vi "Angle Vector to Rotation Matrix.vi"(1 "vector":dbl[](array[numeric]), 2 "angle":dbl) -> (0 "rotation matrix":dbl[][](array[numeric]))   [LabVIEW 2021]
doc: "This VI transforms angle vector to rotation matrix."
uses:
  <vilib>/Analysis/_algsub.llb/Real Vector Norm.vi
  <vilib>/Analysis/baseanly.llb/Real Outer Product.vi
  <vilib>/Analysis/7linalg.llb/Create Special Real Matrix.vi
  <vilib>/Analysis/Matrix/Numeric/Multiply/Multiply - RM,R.vi
  <vilib>/Analysis/Matrix/Numeric/Multiply/Multiply - R,RM.vi
  <vilib>/Analysis/Matrix/Numeric/Add/Add - RM,RM.vi
  <vilib>/Analysis/NI_AALPro.lvlib
  <vilib>/Analysis/NI_AALBase.lvlib
  <vilib>/Analysis/Matrix/NI_Matrix.lvlib
panel:
  # "This VI transforms angle vector to rotation matrix."
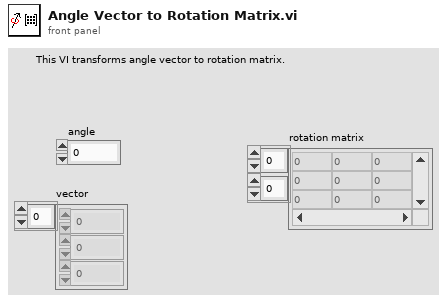
[diagram p1: front panel]
types:
  T1 = enum32{"Identity", "Diagonal", "Toepliz", "Vandermonde", "Companion"}
  T2 = typedef "NI_Matrix.lvlib/RealMatrix.ctl" = dbl[][]
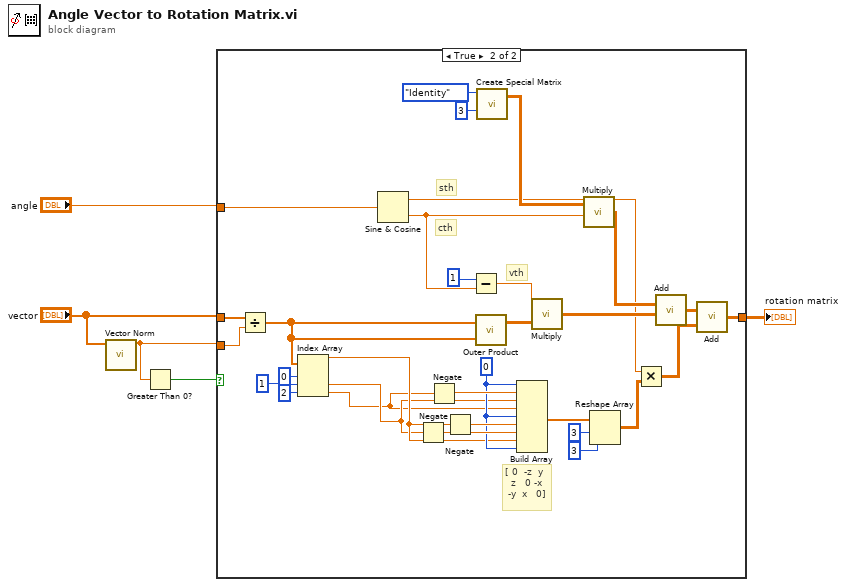
[diagram p0: block diagram]
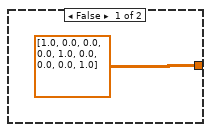
[diagram p2: hidden frame]
diagram:
  n1 = call-poly <vilib>:"Vector Norm.vi"("Input Vector"="vector") -> ("norm"=w2:dbl)  [unwired: 2 in, 8 out]
  n2 = Greater Than 0?(x=w2) -> (x > 0?=w3:bool)
  n3 = case shown="True" w3 {
    tunnel: [dbl[][] [[1.0, 0.0, 0.0], [0.0, 1.0, 0.0], [0.0, 0.0, 1.0]] w28] -> w1
    tunnel: w2 -> [_ w26]
    tunnel: "vector" -> [_ w25]
    tunnel: "angle" -> [_ w22]
    frame False {
    }
    frame True {
      w11 = 0 ("index")
      # "vth"
      # "cth"
      # "sth"
      # "[ 0  -z  y\n  z   0 -x\n -y  x   0]"
      n4 = Divide(x=w25, y=w26) -> (x/y=w18:dbl[])
      n5 = Index Array(array=w18, index #1=0 ("index"), index #2=1 ("index"), index #3=2 ("index")) -> (element #1=w9:dbl, element #2=w8:dbl, element #3=w7:dbl)
      n6 = Sine & Cosine(0:w22) -> (1:w23:dbl, 2:w24:dbl)
      n7 = Negate(x=w8) -> (-x=w14:dbl)
      n8 = Negate(x=w7) -> (-x=w15:dbl)
      n9 = Negate(x=w9) -> (-x=w13:dbl)
      n10 = Subtract(x=1, y=w24) -> (x-y=w36:dbl)
      n11 = call-poly <vilib>:"Outer Product.vi"("Y Vector"=w18, "X Vector"=w18) -> ("Outer Product"=w32:T2)  [unwired: 1 out]
      n12 = call-poly <vilib>:"Create Special Matrix.vi"("matrix type"=T1."Identity", "matrix size"=3) -> ("Special Matrix"=w33:T2)  [unwired: 2 in, 2 out]
      n13 = Build Array(w11, w15, w8, w7, w11, w13, w14, w9, w11) -> (w12:dbl[])
      n14 = call-poly <vilib>:"Multiply.vi"("Real Matrix A"=w32, "Real Scalar c"=w36) -> ("c * A"=w30:T2)
      n15 = call-poly <vilib>:"Multiply.vi"("Real Scalar c"=w24, "Real Matrix A"=w33) -> ("A * c"=w31:T2)
      n16 = Reshape Array(w12, 3 ("dimension size"), 3 ("dimension size")) -> (w10:dbl[][])
      n17 = Multiply ("Multiply.vi")(x=w23, y=w10) -> (x*y=w27:dbl[][])
      n18 = call-poly <vilib>:"Add.vi"("Real Matrix B"=w30, "Real Matrix A"=w31) -> ("A + B"=w29:T2)
      n19 = call-poly <vilib>:"Add.vi"("Real Matrix B"=w27, "Real Matrix A"=w29) -> ("A + B"=w28:T2)
    }
  }
  "rotation matrix" <- w1
